vi "MoveTail.vi"(8 "error in (no error)":errorcluster, 11 "Game Data in":T1) -> (0 "error out":errorcluster, 3 "Game Data out":T1)   [LabVIEW 2020]
uses:
  TypeDef/game-data.ctl
  TypeDef/tiles-key.ctl
  TypeDef/direction.ctl
  <vilib>/Utility/error.llb/Error Cluster From Error Code.vi
  <vilib>/ErrorRing/Error Ring.xnode
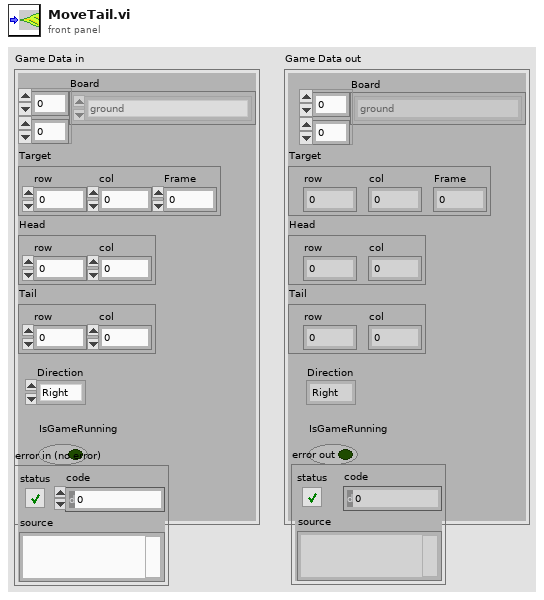
[diagram p1: front panel]
types:
  T1 = typedef "game-data.ctl" = cluster{"Board":T2[][], "Target":cluster{"row":i32, "col":i32, "Frame":i8}, "Head":cluster{"row":i32, "col":i32}, "Tail":cluster{"row":i32, "col":i32}, "Direction":T3, "IsGameRunning":bool, "Points":i32}
  T2 = typedef "tiles-key.ctl" = enum16{"ground", "wall", "head (right)", "head (up)", "head (left)", "head (down)", "L-turn (right-up)", "L-turn (up-left)", "L-turn (left-down)", "L-turn (down-right)", "body (right)", "body (up)", "body (left)", "body (down)", "R-turn (right-down)", "R-turn (up-right)", "R-turn (left-up)", "R-turn (down-left)", "tail (right)", "tail (up)", "tail (left)", "tail (down)", "dead head (right)", "dead head (up)", "dead head (left)", "dead head (down)", "dead L-turn (right-up)", "dead L-turn (up-left)", "dead L-turn (left-down)", "dead L-turn (down-right)", "dead body (right)", "dead body (up)", "dead body (left)", "dead body (down)", "dead R-turn (right-down)", "dead R-turn (up-right)", "dead R-turn (left-up)", "dead R-turn (down-left)", "dead tail (right)", "dead tail (up)", "dead tail (left)", "dead tail (down)", "target red", "target blue", "target yellow", "target green"}
  T3 = typedef "direction.ctl" = enum16{"Right", "Up", "Left", "Down"}
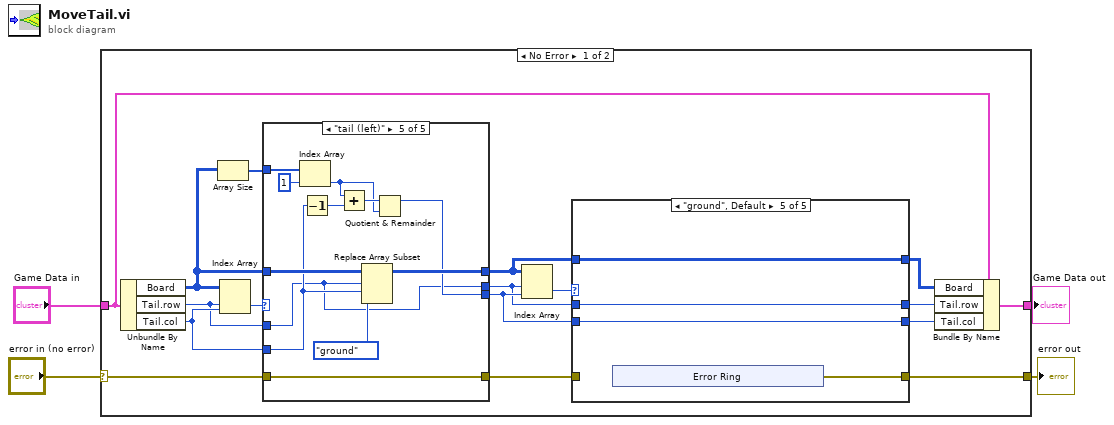
[diagram p0: block diagram]
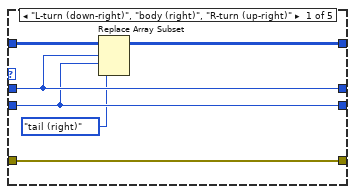
[diagram p2: hidden frame]
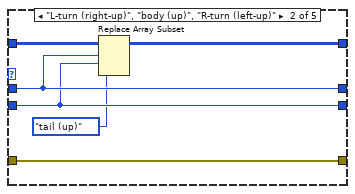
[diagram p3: hidden frame]
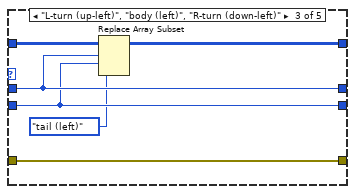
[diagram p4: hidden frame]
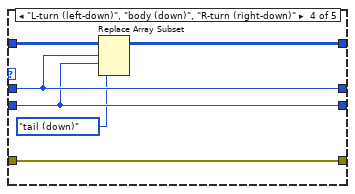
[diagram p5: hidden frame]
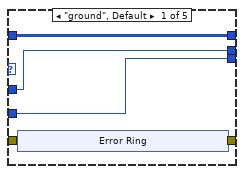
[diagram p6: hidden frame]
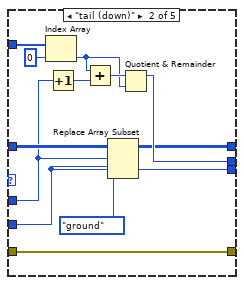
[diagram p7: hidden frame]
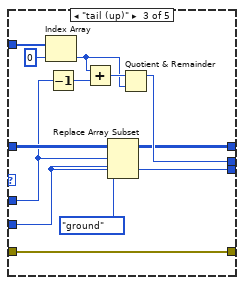
[diagram p8: hidden frame]
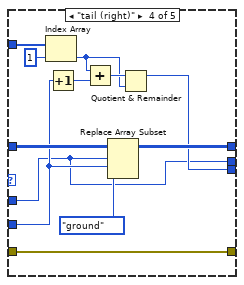
[diagram p9: hidden frame]
diagram:
  n1 = case shown="No Error" "error in (no error)" {
    selector: "error in (no error)" -> [w18 w113]
    tunnel: [w5 w113] -> w3
    tunnel: "Game Data in" -> [w20 w112]
    tunnel: [w21 w112] -> w1
    frame No Error {
      n2 = Unbundle By Name(w20) -> ("Board"=w14:T2[][], "Tail.row"=w15:i32, "Tail.col"=w16:i32)
      n3 = Array Size(array=w14) -> (size(s)=w17:i32[])
      n4 = Index Array(array=w14, index (row)=w15, index (col)=w16) -> (element=w19:T2)
      n5 = case shown="\"tail (left)\"" w19 {
        tunnel: w18 -> [_ w75 w87 w99 w111]
        tunnel: [w58 w75 w87 w99 w111] -> w6
        tunnel: w17 -> [_ w72 w84 w96 w108]
        tunnel: w16 -> [w55 w65 w77 w89 w101]
        tunnel: w15 -> [w56 w68 w80 w88 w100]
        tunnel: w14 -> [w57 w74 w86 w98 w110]
        tunnel: [w56 w66 w78 w88 w100] -> w8
        tunnel: [w55 w65 w77 w90 w102] -> w9
        tunnel: [w57 w64 w76 w91 w103] -> w12
        frame "ground", Default {
          n6 = xnode "Error Ring"() -> ("error out"=w58:errorcluster)
        }
        frame "tail (down)" {
          n7 = Index Array(array=w72, index=0) -> (element=w69:i32)
          n8 = Increment(x=w68) -> (x+1=w67:i32)
          n9 = Add(x=w69, y=w67) -> (x+y=w70:i32)
          n10 = Replace Array Subset(array=w74, new element=tiles-key."ground" ("new element/subarray"), index (row)=w68, index (col)=w65) -> (w64:T2[][])
          n11 = Quotient & Remainder(x=w70, y=w69) -> (x-y*floor(x/y)=w66:i32)  [unwired: 1 out]
        }
        frame "tail (up)" {
          n12 = Index Array(array=w84, index=0) -> (element=w81:i32)
          n13 = Decrement(x=w80) -> (x-1=w79:i32)
          n14 = Add(x=w81, y=w79) -> (x+y=w82:i32)
          n15 = Replace Array Subset(array=w86, new element=tiles-key."ground" ("new element/subarray"), index (row)=w80, index (col)=w77) -> (w76:T2[][])
          n16 = Quotient & Remainder(x=w82, y=w81) -> (x-y*floor(x/y)=w78:i32)  [unwired: 1 out]
        }
        frame "tail (right)" {
          n17 = Index Array(array=w96, index=1) -> (element=w93:i32)
          n18 = Increment(x=w89) -> (x+1=w92:i32)
          n19 = Add(x=w93, y=w92) -> (x+y=w94:i32)
          n20 = Replace Array Subset(array=w98, new element=tiles-key."ground" ("new element/subarray"), index (row)=w88, index (col)=w89) -> (w91:T2[][])
          n21 = Quotient & Remainder(x=w94, y=w93) -> (x-y*floor(x/y)=w90:i32)  [unwired: 1 out]
        }
        frame "tail (left)" {
          n22 = Index Array(array=w108, index=1) -> (element=w105:i32)
          n23 = Decrement(x=w101) -> (x-1=w104:i32)
          n24 = Add(x=w105, y=w104) -> (x+y=w106:i32)
          n25 = Replace Array Subset(array=w110, new element=tiles-key."ground" ("new element/subarray"), index (row)=w100, index (col)=w101) -> (w103:T2[][])
          n26 = Quotient & Remainder(x=w106, y=w105) -> (x-y*floor(x/y)=w102:i32)  [unwired: 1 out]
        }
      }
      n27 = Index Array(array=w12, index (row)=w8, index (col)=w9) -> (element=w13:T2)
      n28 = case shown="\"ground\", Default" w13 {
        tunnel: w12 -> [w27 w33 w39 w45 w46]
        tunnel: [w26 w32 w38 w44 w46] -> w11
        tunnel: [w24 w30 w36 w42 w48] -> w10
        tunnel: w9 -> [w24 w30 w36 w42 w48]
        tunnel: w8 -> [w25 w31 w37 w43 w47]
        tunnel: [w25 w31 w37 w43 w47] -> w7
        tunnel: w6 -> [w22 w28 w34 w40 _]
        tunnel: [w22 w28 w34 w40 w49] -> w5
        frame "L-turn (down-right)", "body (right)", "R-turn (up-right)" {
          n29 = Replace Array Subset(array=w27, new element=tiles-key."tail (right)" ("element"), index (row)=w25, index (col)=w24) -> (w26:T2[][])
        }
        frame "L-turn (right-up)", "body (up)", "R-turn (left-up)" {
          n30 = Replace Array Subset(array=w33, new element=tiles-key."tail (up)" ("element"), index (row)=w31, index (col)=w30) -> (w32:T2[][])
        }
        frame "L-turn (up-left)", "body (left)", "R-turn (down-left)" {
          n31 = Replace Array Subset(array=w39, new element=tiles-key."tail (left)" ("element"), index (row)=w37, index (col)=w36) -> (w38:T2[][])
        }
        frame "L-turn (left-down)", "body (down)", "R-turn (right-down)" {
          n32 = Replace Array Subset(array=w45, new element=tiles-key."tail (down)" ("element"), index (row)=w43, index (col)=w42) -> (w44:T2[][])
        }
        frame "ground", Default {
          n33 = xnode "Error Ring"() -> ("error out"=w49:errorcluster)
        }
      }
      n34 = Bundle By Name(cluster=w20, "Board"=w11, "Tail.row"=w7, "Tail.col"=w10) -> (w21:T1)
    }
    frame Error {
    }
  }
  "Game Data out" <- w1
  "error out" <- w3
